vi "Abort.vi"(8 "error in (no error)":errorcluster, 11 "Object ref in":T1) -> (0 "error out":errorcluster, 3 "Object ref out":T1)   [LabVIEW 2013, in "PowderDeposition.lvlib" / "PD-Main.lvclass"]
uses:
  PD-Main.lvclass
  Object-reference.ctl
  Client-status.ctl
  PD-Main.lvclass/PD-Main.ctl
  Assembly/Motor-assembly.lvclass
  Motor/Motor.lvclass
  Read Motor assembly.vi
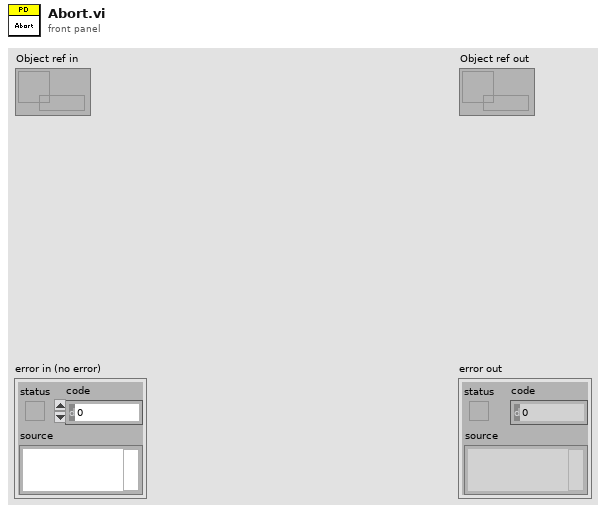
[diagram p1: front panel]
types:
  T1 = typedef "PowderDeposition.lvlib/PD-Main.lvclass/Object-reference.ctl" = refnum<data-value>
  T2 = typedef "PowderDeposition.lvlib/PD-Main.lvclass/Client-status.ctl" = enum16{"Idle", "Initialized", "Configured", "Activated", "Started", "Paused", "Stopped", "Reset", "Error", "Exited"}
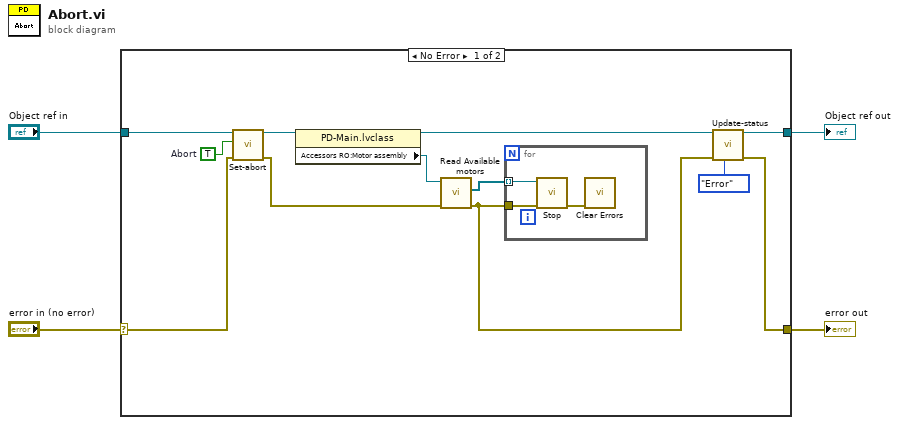
[diagram p0: block diagram]
diagram:
  n1 = case shown="No Error" "error in (no error)" {
    selector: "error in (no error)" -> [w11 w21]
    tunnel: [w6 w21] -> w3
    tunnel: [w5 w20] -> w1
    tunnel: "Object ref in" -> [w15 w20]
    frame No Error {
      w16 = TRUE  # Abort
      n2 = call "Set-abort.vi"("error in (no error)"=w11, "Abort"=w16, "Object ref in"=w15) -> ("error out"=w10:errorcluster, "Object ref out"=w14:T1)  [unwired: 7 in]
      n3 = property class="PD-Main.lvclass"(reference=w14) -> (reference out=w8:T1, "Accessors RO:Motor assembly"=w12:refnum<class "Motor-assembly.lvclass">)  [unwired: 1 in, 1 out]
      n4 = call-dynamic "Read Available motors.vi"("error in (no error)"=w10, "Available motors in"=w12) -> ("error out"=w7:errorcluster, "Available motors"=w13:refnum<class "Motor.lvclass">[])  [unwired: 7 in, 1 out]
      n5 = for {
        tunnel: w13 -> [w19] mode=indexing
        tunnel: w7 -> [w18]
        n6 = call-dynamic "Stop.vi"("error in (no error)"=w18, "Motor in"=w19) -> ("error out"=w17:errorcluster)  [unwired: 8 in, 1 out]
        n7 = call <vilib>:"Clear Errors.vi"("error in (no error)"=w17) -> ()  [unwired: 6 in, 1 out]
      }
      n8 = call "Update-status.vi"("Status"=Client-status."Error", "error in (no error)"=w7, "Object ref in"=w8) -> ("error out"=w6:errorcluster, "Object ref out"=w5:T1)  [unwired: 7 in]
    }
    frame Error {
    }
  }
  "error out" <- w3
  "Object ref out" <- w1
